vi "blcontrol.vi"() -> ()   [LabVIEW 2015]
uses:
  <vilib>/Utility/error.llb/whitespace.ctl
  <vilib>/Instr/_visa.llb/VISA Configure Serial Port (Instr).vi
  passing_instructions/bin/Debug/passing_instructions.dll
panel:
  out "Ready?":bool
  in  "Stop":bool
  out "read buffer":string
  in  "Bluetooth receive port":refnum<visa-resource-name>
  in  "Bluetooth send port":refnum<visa-resource-name>
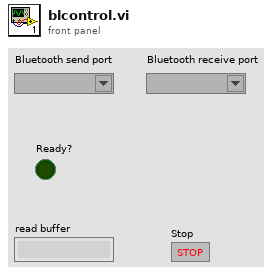
[diagram p1: front panel]
types:
  T1 = typedef "whitespace.ctl" = u16
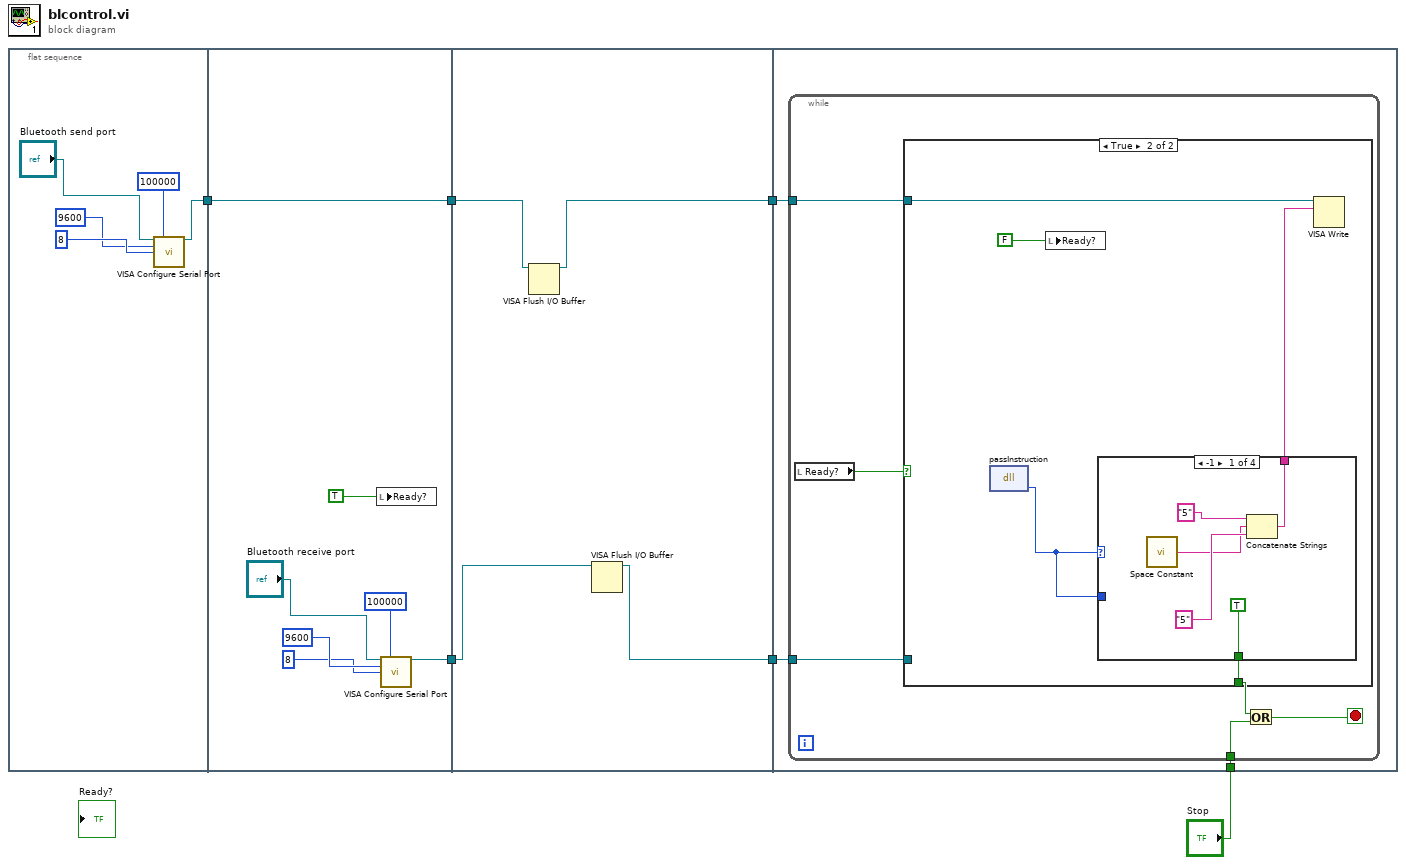
[diagram p0: block diagram]
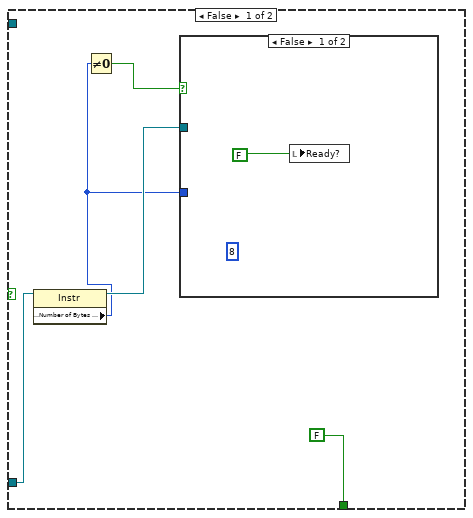
[diagram p2: hidden frame]
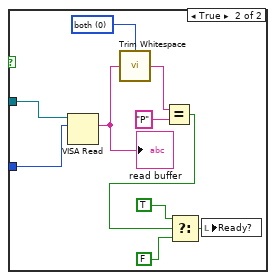
[diagram p3: hidden frame]
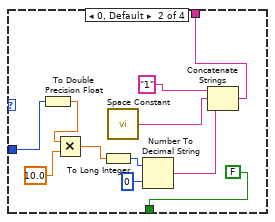
[diagram p4: hidden frame]
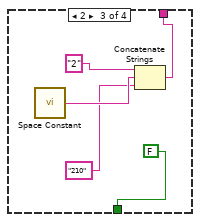
[diagram p5: hidden frame]
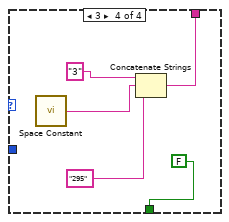
[diagram p6: hidden frame]
diagram:
  n1 = flat-sequence {
    tunnel: [w7] -> w6
    tunnel: [w12] -> w5
    tunnel: [w13] -> w3
    tunnel: w6 -> [w12]
    tunnel: w5 -> [w22]
    tunnel: [w21] -> w4
    tunnel: w3 -> [w20]
    tunnel: [w19] -> w2
    tunnel: w4 -> [w25]
    tunnel: w2 -> [w24]
    tunnel: "Stop" -> [w23]
    frame #0 {
      n2 = call-poly "VISA Configure Serial Port"("VISA resource name"="Bluetooth send port", "timeout (10sec)"=u32 100000, "baud rate (9600)"=u32 9600, "data bits (8)"=u16 8) -> ("VISA resource name out"=w7:refnum<visa-resource-name>)  [unwired: 10 in, 1 out]
    }
    frame #1 {
      n3 = local write "Ready?"(TRUE) -> ()
      n4 = call-poly "VISA Configure Serial Port"("VISA resource name"="Bluetooth receive port", "timeout (10sec)"=u32 100000, "baud rate (9600)"=u32 9600, "data bits (8)"=u16 8) -> ("VISA resource name out"=w13:refnum<visa-resource-name>)  [unwired: 10 in, 1 out]
    }
    frame #2 {
      n5 = VISA Flush I/O Buffer(VISA resource name=w22) -> (VISA resource name out=w21:refnum<visa-resource-name>)  [unwired: 2 in, 1 out]
      n6 = VISA Flush I/O Buffer(VISA resource name=w20) -> (VISA resource name out=w19:refnum<visa-resource-name>)  [unwired: 2 in, 1 out]
    }
    frame #3 {
      n7 = while {
        tunnel: w25 -> [w31]
        tunnel: w24 -> [w29]
        tunnel: w23 -> [w27]
        stop <- w28 stop-if-true
        n8 = local read "Ready?"() -> (w30:bool)
        n9 = case shown="True" w30 {
          tunnel: w31 -> [_ w52]
          tunnel: w29 -> [w36 _]
          tunnel: [FALSE w48] -> w26
          frame False {
            (unwired) u32 8 ("byte count")
            n10 = property class="Instr"(reference=w36) -> (reference out=w34:refnum<visa-resource-name>, "Serial Settings:Number of Bytes at Serial Port"=w33:u32)  [unwired: 1 in, 1 out]
            n11 = Not Equal To 0?(x=w33) -> (x != 0?=w35:bool)
            n12 = case shown="False" w35 {
              tunnel: w34 -> [_ w39]
              tunnel: w33 -> [_ w38]
              frame False {
                n13 = local write "Ready?"(FALSE) -> ()
              }
              frame True {
                w40 = T1 0 items=["both", "start of string", "end of string"] ("location (both)")
                n14 = VISA Read(VISA resource name=w39, byte count=w38) -> (read buffer=w41:string)  [unwired: 1 in, 3 out]
                "read buffer" <- w41
                n15 = call <vilib>:"Trim Whitespace.vi"("string"=w41, "location (both)"=w40) -> ("trimmed string"=w42:string)
                n16 = Equal?(x=w42, y="P") -> (x = y?=w44:bool)
                n17 = Select(t=TRUE, s=w44, f=FALSE) -> (s? t:f=w47:bool)
                n18 = local write "Ready?"(w47) -> ()
              }
            }
          }
          frame True {
            n19 = dll-call lib="C:/Users/RaduMatei/Desktop/passing_instructions/bin/Debug/passing_instructions.dll" fn="passInstruction"() -> ("return type"=w51:i32)  [unwired: 3 in, 2 out]
            n20 = local write "Ready?"(FALSE) -> ()
            n21 = case shown="-1" w51 {
              tunnel: w51 -> [_ w60 _ _]
              tunnel: [w54 w64 w71 w76] -> w50
              tunnel: [TRUE FALSE FALSE FALSE] -> w48
              frame -1 {
                n22 = call <vilib>:"Space Constant.vi"() -> ("String"=w55:string)
                n23 = Concatenate Strings("5", w55, "5") -> (w54:string)
              }
              frame 0, Default {
                n24 = To Double Precision Float(number=w60) -> (double precision float=w61:dbl)
                n25 = Multiply(x=w61, y=10.0) -> (x*y=w62:dbl)
                n26 = To Long Integer(number=w62) -> (32bit integer=w63:i32)
                n27 = call <vilib>:"Space Constant.vi"() -> ("String"=w67:string)
                n28 = Number To Decimal String(number=w63, width (-)=i16 0) -> (decimal integer string=w65:string)
                n29 = Concatenate Strings("1", w67, w65) -> (w64:string)
              }
              frame 2 {
                n30 = call <vilib>:"Space Constant.vi"() -> ("String"=w73:string)
                n31 = Concatenate Strings("2", w73, "210") -> (w71:string)
              }
              frame 3 {
                n32 = call <vilib>:"Space Constant.vi"() -> ("String"=w78:string)
                n33 = Concatenate Strings("3", w78, "295") -> (w76:string)
              }
            }
            n34 = VISA Write(VISA resource name=w52, write buffer=w50) -> ()  [unwired: 1 in, 3 out]
          }
        }
        n35 = Or(x=w26, y=w27) -> (x .or. y?=w28:bool)
      }
    }
  }
